vi "Read stop event.vi"(8 "error in (no error)":errorcluster, 11 "Measure Object in":refnum<class "Da Base.lvclass">) -> (0 "error out":errorcluster, 2 "stop event":refnum<user-event>, 3 "Measure Object out":refnum<class "Da Base.lvclass">)   [LabVIEW 2016, in "Da Base.lvclass"]
uses:
  Da Base.lvclass
  Da Base.lvclass/Da Base.ctl
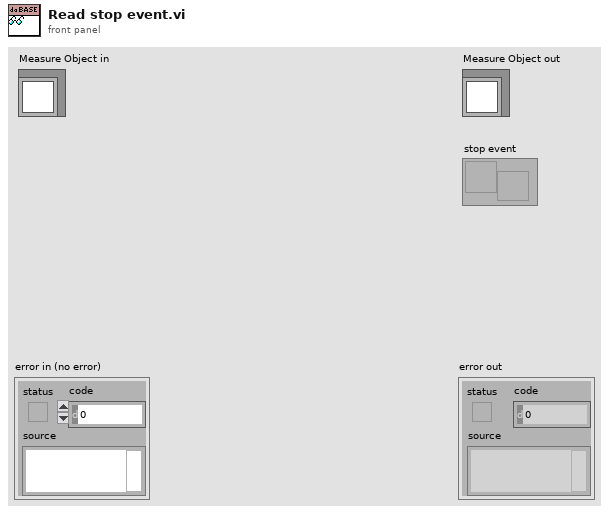
[diagram p1: front panel]
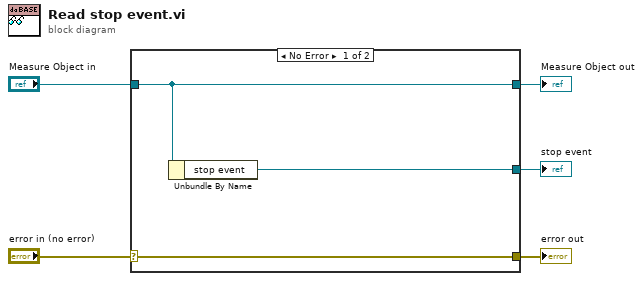
[diagram p0: block diagram]
diagram:
  n1 = case shown="No Error" "error in (no error)" {
    selector: "error in (no error)" -> [w8 w9]
    tunnel: [w8 w9] -> w4
    tunnel: [w7 w10] -> w2
    tunnel: "Measure Object in" -> [w7 w10]
    tunnel: [w6 _] -> w1
    frame No Error {
      n2 = Unbundle By Name(w7) -> ("stop event"=w6:refnum<user-event>)
    }
    frame Error {
    }
  }
  "error out" <- w4
  "Measure Object out" <- w2
  "stop event" <- w1
